vi "Status Info Read.vi"(8 "error in (no error)":errorcluster, 11 "RT data in":T1) -> (0 "error out":errorcluster, 3 "RT data out":T1)   [LabVIEW 2011, in "Engine Sim RT.lvlib"]
uses:
  Engine Sim RT.lvlib
  TypeDefs/RT Data Cluster.ctl
  Shared/Channel Descriptors.ctl
  Shared/FPGA Write Descriptor.ctl
  Shared/InputChannelTypes.ctl
  <vilib>/rvi/DataTransferAndStorage/Container/Common/niFpgaDataTypeControl.ctl
  Shared/FPGA Read Descriptor.ctl
  Shared/OutputChannelTypes.ctl
  Shared/Status Chan Descriptor.ctl
  Shared/DataReplayVoltageConfig.ctl
  Engine Simulation Shared.lvlib
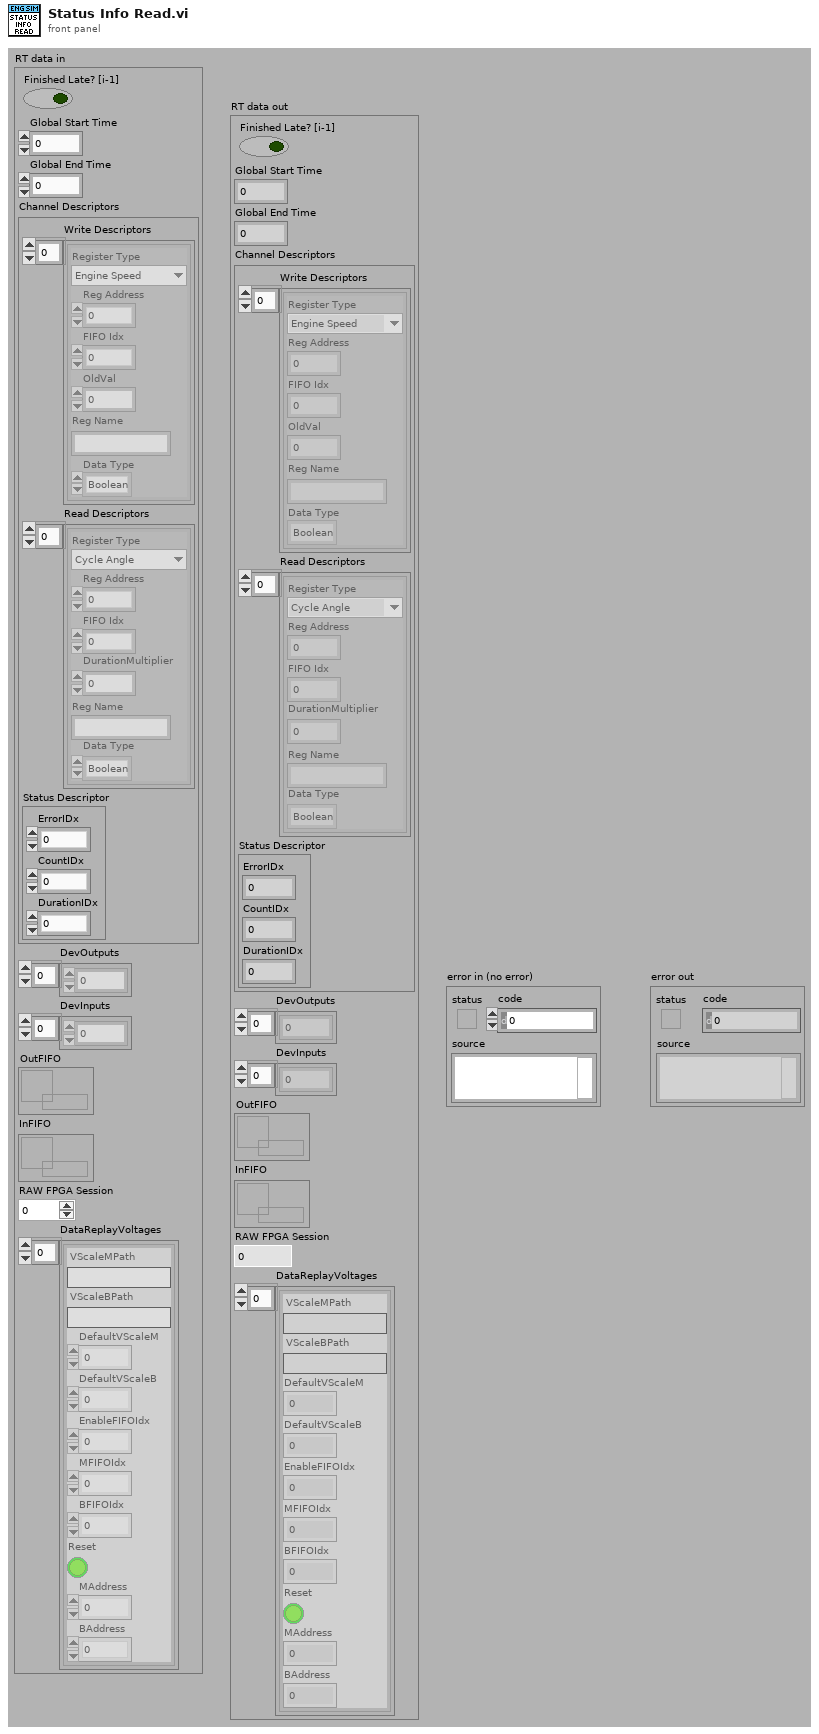
[diagram p1: front panel]
types:
  T1 = typedef "Engine Sim RT.lvlib/RT Data Cluster.ctl" = cluster{"Finished Late? [i-1]":bool, "Global Start Time":i64, "Global End Time":i64, "Channel Descriptors":T2, "DevOutputs":dbl[], "DevInputs":dbl[], "OutFIFO":refnum<k33>, "InFIFO":refnum<k33>, "RAW FPGA Session":u32, "DataReplayVoltages":T9[]}
  T2 = typedef "Engine Simulation Shared.lvlib/Channel Descriptors.ctl" = cluster{"Write Descriptors":T3[], "Read Descriptors":T6[], "Status Descriptor":T8}
  T3 = typedef "Engine Simulation Shared.lvlib/FPGA Write Descriptor.ctl" = cluster{"Register Type":T4, "Reg Address":u32, "FIFO Idx":i32, "OldVal":dbl, "Reg Name":string, "Data Type":T5}
  T4 = typedef "Engine Simulation Shared.lvlib/InputChannelTypes.ctl" = enum16{"Engine Speed", "Offset"}
  T5 = typedef "niFpgaDataTypeControl.ctl" = enum32{"Boolean", "I8", "I16", "I32", "I64", "U8", "U16", "U32", "U64", "FXP", "CustomControl"}
  T6 = typedef "Engine Simulation Shared.lvlib/FPGA Read Descriptor.ctl" = cluster{"Register Type":T7, "Reg Address":u32, "FIFO Idx":i32, "DurationMultiplier":dbl, "Reg Name":string, "Data Type":T5}
  T7 = typedef "Engine Simulation Shared.lvlib/OutputChannelTypes.ctl" = enum16{"Cycle Angle", "Crank Angle", "Time Duration", "Angle Duration", "Start Angle", "End Angle"}
  T8 = typedef "Engine Simulation Shared.lvlib/Status Chan Descriptor.ctl" = cluster{"ErrorIDx":i32, "CountIDx":i32, "DurationIDx":i32}
  T9 = typedef "Engine Simulation Shared.lvlib/DataReplayVoltageConfig.ctl" = cluster{"VScaleMPath":string, "VScaleBPath":string, "DefaultVScaleM":u32, "DefaultVScaleB":i32, "EnableFIFOIdx":i32, "MFIFOIdx":i32, "BFIFOIdx":i32, "Reset":bool, "MAddress":u32, "BAddress":u32}
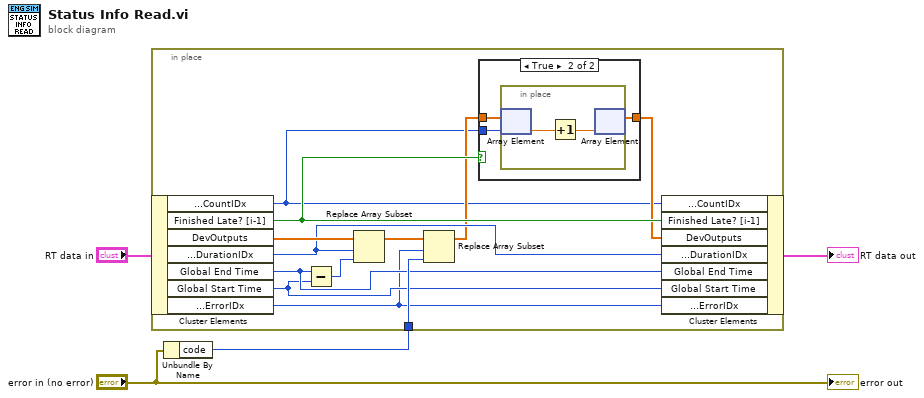
[diagram p0: block diagram]
diagram:
  n1 = Unbundle By Name("error in (no error)") -> ("code"=w2:i32)
  n2 = in-place {
    in-place-border: w2 -> [w13]
    n3 = in-place-cluster #1("RT data in") -> ("Channel Descriptors.Status Descriptor.CountIDx"=w5:i32, "Finished Late? [i-1]"=w8:bool, "DevOutputs"=w16:dbl[], "Channel Descriptors.Status Descriptor.DurationIDx"=w12:i32, "Global End Time"=w11:i64, "Global Start Time"=w10:i64, "Channel Descriptors.Status Descriptor.ErrorIDx"=w9:i32)
    n4 = Subtract(x=w11, y=w10) -> (x-y=w15:i64)
    n5 = Replace Array Subset(array=w16, new element=w15, index=w12) -> (w14:dbl[])
    n6 = Replace Array Subset(array=w14, new element=w13, index=w9) -> (w7:dbl[])
    n7 = case shown="True" w8 {
      tunnel: w7 -> [w17 w20]
      tunnel: [w17 w19] -> w6
      tunnel: w5 -> [_ w18]
      frame False {
      }
      frame True {
        n8 = in-place {
          n9 = in-place-array #2(w20, w18) -> (w22:dbl)
          n10 = Increment(x=w22) -> (x+1=w21:dbl)
          n11 = in-place-array #2(w21) -> (w19:dbl[])  [unwired: 1 out]
        }
      }
    }
    n12 = in-place-cluster #1("Channel Descriptors.Status Descriptor.CountIDx"=w5, "Finished Late? [i-1]"=w8, "DevOutputs"=w6, "Channel Descriptors.Status Descriptor.DurationIDx"=w12, "Global End Time"=w11, "Global Start Time"=w10, "Channel Descriptors.Status Descriptor.ErrorIDx"=w9) -> (→"RT data out":T1)
  }
  "error out" <- "error in (no error)"
